vi "Accelerator_v2.002_small.vi"() -> ()   [LabVIEW 2013]
doc: "Acquire Accelerator Data"
uses:
  <instrlib>/niScope/Controls/niScope vertical coupling.ctl
  <instrlib>/niScope/Controls/niScope trigger slope.ctl
  <instrlib>/niScope/Controls/niScope trigger coupling.ctl
  <instrlib>/niScope/Controls/niScope trigger source.ctl
  Accelerator Measurement/Array_Defctl.ctl
  <vilib>/Utility/error.llb/DialogType.ctl
  <vilib>/Utility/miscctls.llb/LVPointTypeDef.ctl
  <vilib>/Utility/miscctls.llb/LVPositionTypeDef.ctl
  Public API/Dust_Event.ctl
  Public API/Signal.ctl
  Private/Role ID.ctl
  Private/Hardware ID.ctl
  Private/Estimate_source.ctl
  Functional Global Variables/Action Items.ctl
  <vilib>/Analysis/baseanly.llb/Mean (DBL).vi
  Private/PSU updated.vi
  <vilib>/addons/database/Connection.llb/Conn Execute.vi
  <vilib>/addons/database/Recordset.llb/Rec Fetch Recordset Data (R).vi
  <vilib>/addons/database/Recordset.llb/Rec Destroy - Connection.vi
  <instrlib>/niScope/Configure/Trigger/niScope Configure Trigger Edge.vi
  <instrlib>/niScope/Acquire/Fetch/niScope Multi Fetch Cluster.vi
  <vilib>/addons/database/_DB Variant To Data/Database Variant To Data.xnode
  <vilib>/Analysis/NI_AALBase.lvlib
  <vilib>/addons/database/NI_Database_API.lvlib
panel:
  in  "Trigger":enum32{"Edge"}(tab)
  in  "Trigger Source Edge 2":T1="2" caption="Source"
  in  "Trigger Source Edge":T1="0" caption="Source"
  in  "Coupling":T2=1 items=["AC"=0, "DC"=1, "HF Reject"=3, "LF Reject"=4, "AC Plus HF Reject"=1001]
  in  "Slope":T3 caption="Trigger Slope"
  in  "Level":dbl=1.0 caption="Trigger Level" step=0.001 format="%.3f"
  in  "Delay":dbl caption="Trigger Delay" format="%.4p"
  in  "Reference Position (%)":dbl=40.0 caption="Ref Position" format="%.1f"
  in  "Bandwidth":dbl=-1.0 format="%.2f"
  in  "Vertical Coupling":T4=1 items=["AC", "DC", "Ground"]
  in  "Probe Attenuation":dbl=1.0 format="%.1f"
  in  "Vertical Offset":dbl format="%.4f"
  in  "Vertical Range":dbl=5.0 caption="Vertical Range (V)" format="%.2f"
  out "Actual Sample Rate":dbl=10000000.0 format="%.0p"
  in  "Min Record Length":i32=100000 caption="Min. Record Length"
  in  "Min Sample Rate":dbl=80000000.0 caption="Min. Sample Rate" step=1000000.0 format="%.2p"
  out "Actual Record Length":i32=100000
  out "Mass":dbl format="%#_3g"
  in  "Write to Database?":bool=TRUE
  in  "Limit":dbl
  in  "Limit Triggers":bool
  out "Acquisition #":i32
  in  "WFM Tag":string="trace"
  in  "Location":string="G:\\default"
  in  "Write Raw File?":bool
  out "Saving Raw File...":path=path "G:/2012_06_13_verify_timestamp_labview/trace00000"
  out "?":cluster{dbl, dbl}(knob)={0.0549, 2.0} scale=10.0..0.01
  in  "Ideal Time (Cursor)":dbl=2.0 step=0.01 format="%_2f"
  out "Time Between Triggers":dbl
  out "Average Frequency":dbl format="%#_4g"
  out "output cluster":T5
  out "error out 4":errorcluster
  out "error out 3":errorcluster
  out "# elements in queue":i32
  out "Stop condition":bool=TRUE
  out "created path":path=path "G:/default"
  out "Numeric":i32=92364
  out "error out 2":errorcluster
  out "Calibration":dbl=24700000000000.0
  out "Array":T6=["Dev1", "Dev2"]
  out "Multi Plot 2":cluster{dbl[], dbl[]}(graph) caption="Multi Plot"
  in  "Acceleration Voltage (MV)":dbl=2.0 format="%_2g"
  out "Charge":dbl format="%#_3g"
  out "Velocity (Est.)":dbl format="%#_6f"
  out "Final Detector (CH3)":waveform(dbl)(graph)={"t0"=timestamp(0 s since 1904-01-01), "dt"=1e-07, "Y"=[]}
  out "Charge Detector/PSU gate (CH2)":waveform(dbl)(graph)={"t0"=timestamp(0 s since 1904-01-01), "dt"=1e-07, "Y"=[]}
  out "Velocity Detectors (CH0 & CH1)":waveform(dbl)[](graph)
  in  "stop":bool=TRUE
  out "error out":errorcluster={"status"=FALSE, "code"=0, "source"="No Error"} {"code" format="%.0x"}
  # "File Parameters"
  # "Error Handling"
  # "Trigger"
  # "Channel"
  # "Vertical"
  # "Horizontal"
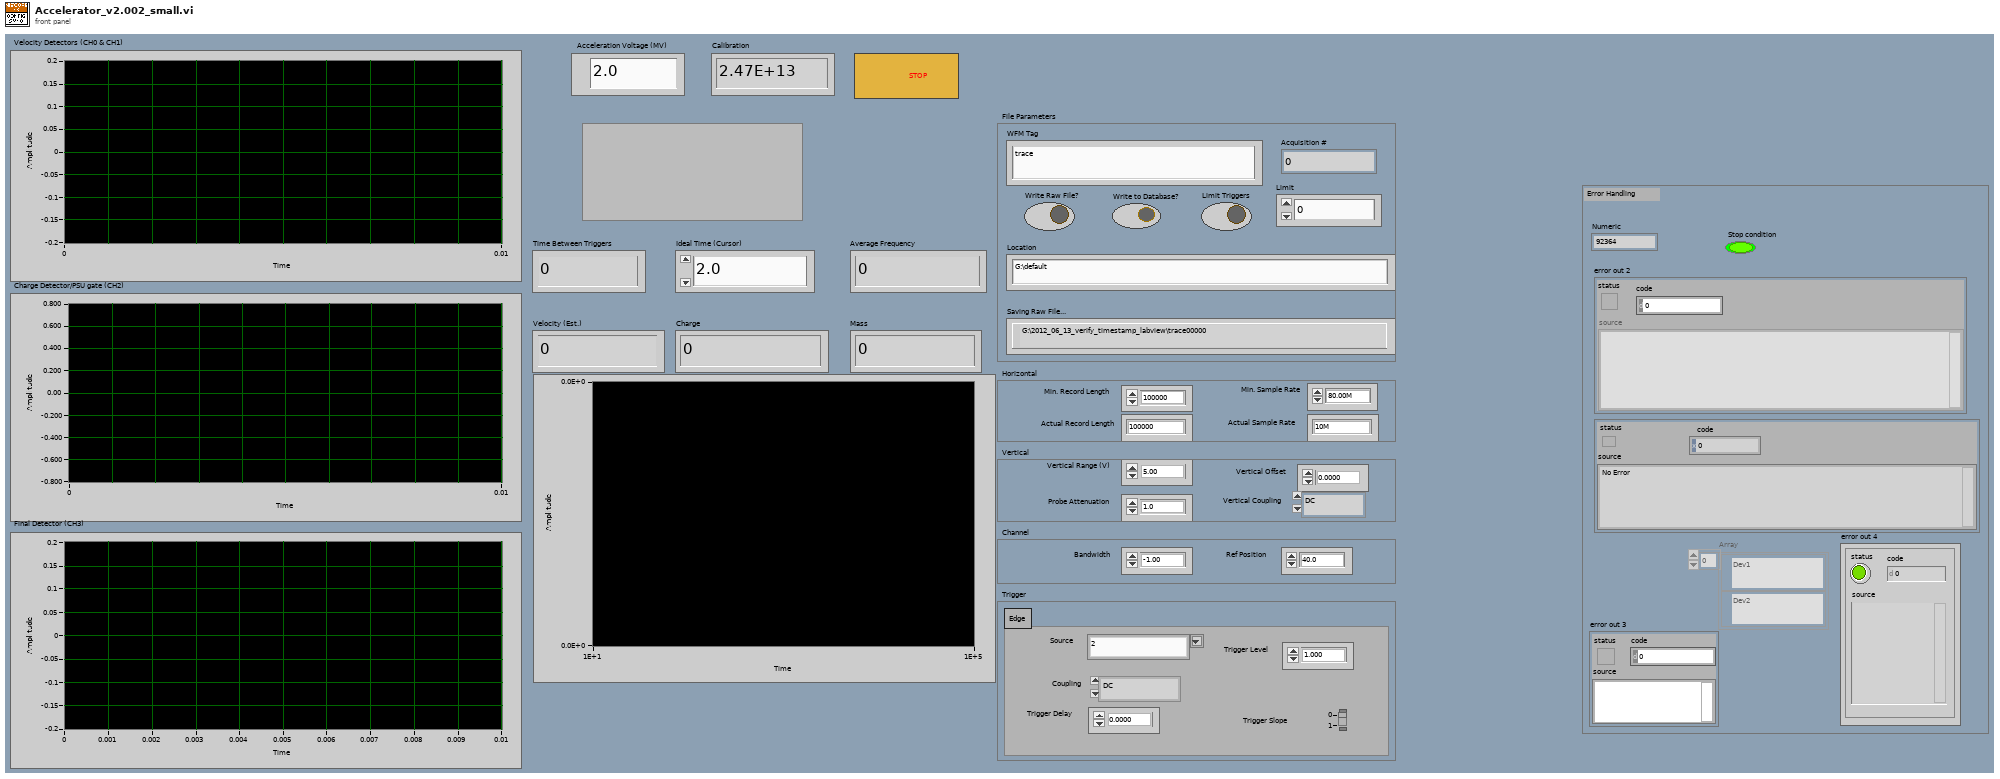
[diagram p1: front panel]
types:
  T1 = typedef "niScope trigger source.ctl" = string
  T2 = typedef "niScope trigger coupling.ctl" = u16
  T3 = typedef "niScope trigger slope.ctl" = i32
  T4 = typedef "niScope vertical coupling.ctl" = i32
  T5 = cluster{"File Path Control":path, "Array":waveform(dbl)[]}
  T6 = typedef "Array_Defctl.ctl" = refnum<k15>[]
  T7 = typedef "LVPointTypeDef.ctl" = cluster{"Horizontal":i16, "Vertical":i16}
  T8 = typedef "DialogType.ctl" = u16
  T9 = typedef "LVPositionTypeDef.ctl" = cluster{"Left":i32, "Top":i32}
  T10 = typedef "NI_Database_API.lvlib/Conn ObjectReference.ctl" = refnum<k1>
  T11 = typedef "NI_Database_API.lvlib/Rec ObjectReference.ctl" = refnum<k1>
  T12 = cluster{"Integer Timestamp":dbl, "Max Velocity":dbl, "Min Velocity":dbl}
  T13 = cluster{"first point time":dbl, "xIncrement":dbl, "Waveforms":dbl[]}[]
  T14 = typedef "Dust_Event.ctl" = cluster{"Time Stamp":timestamp, "Velocity":sgl, "Mass":sgl, "Charge":sgl, "Radius":sgl, "Array":T15[], "Dust Event ID":i64, "Passed_3rd_Detector":bool, "Estimate Source":T18, "Estimate Quality":sgl}
  T15 = typedef "Signal.ctl" = cluster{"Signal ID":i64, "Time Stamp":timestamp, "Dust Event ID":i64, "Role ID":T16, "Data":sgl[], "Signal Length":i32, "dt":sgl, "Offset":dbl, "Hardware ID":T17}
  T16 = typedef "Role ID.ctl" = enum16{"First_Detector", "Second_Detector", "Third_Detector", "LeCroy_CH1", "LeCroy_CH2", "LeCroy_CH3", "LeCroy_CH4", "PSU"}
  T17 = typedef "Hardware ID.ctl" = enum16{"Unknown", "CSA 1", "CSA 2", "CSA 3", "CSA 4", "CSA 5", "CSA 6"}
  T18 = typedef "Estimate_source.ctl" = i8
  T19 = typedef "Action Items.ctl" = enum16{"Initialize", "Get", "Set"}
  T20 = cluster{"relativeInitialX":dbl, "xIncrement":dbl, "wfm":dbl[]}[]
  T21 = cluster{"first point time":dbl, "xIncrement":dbl, "Waveforms":dbl[]}
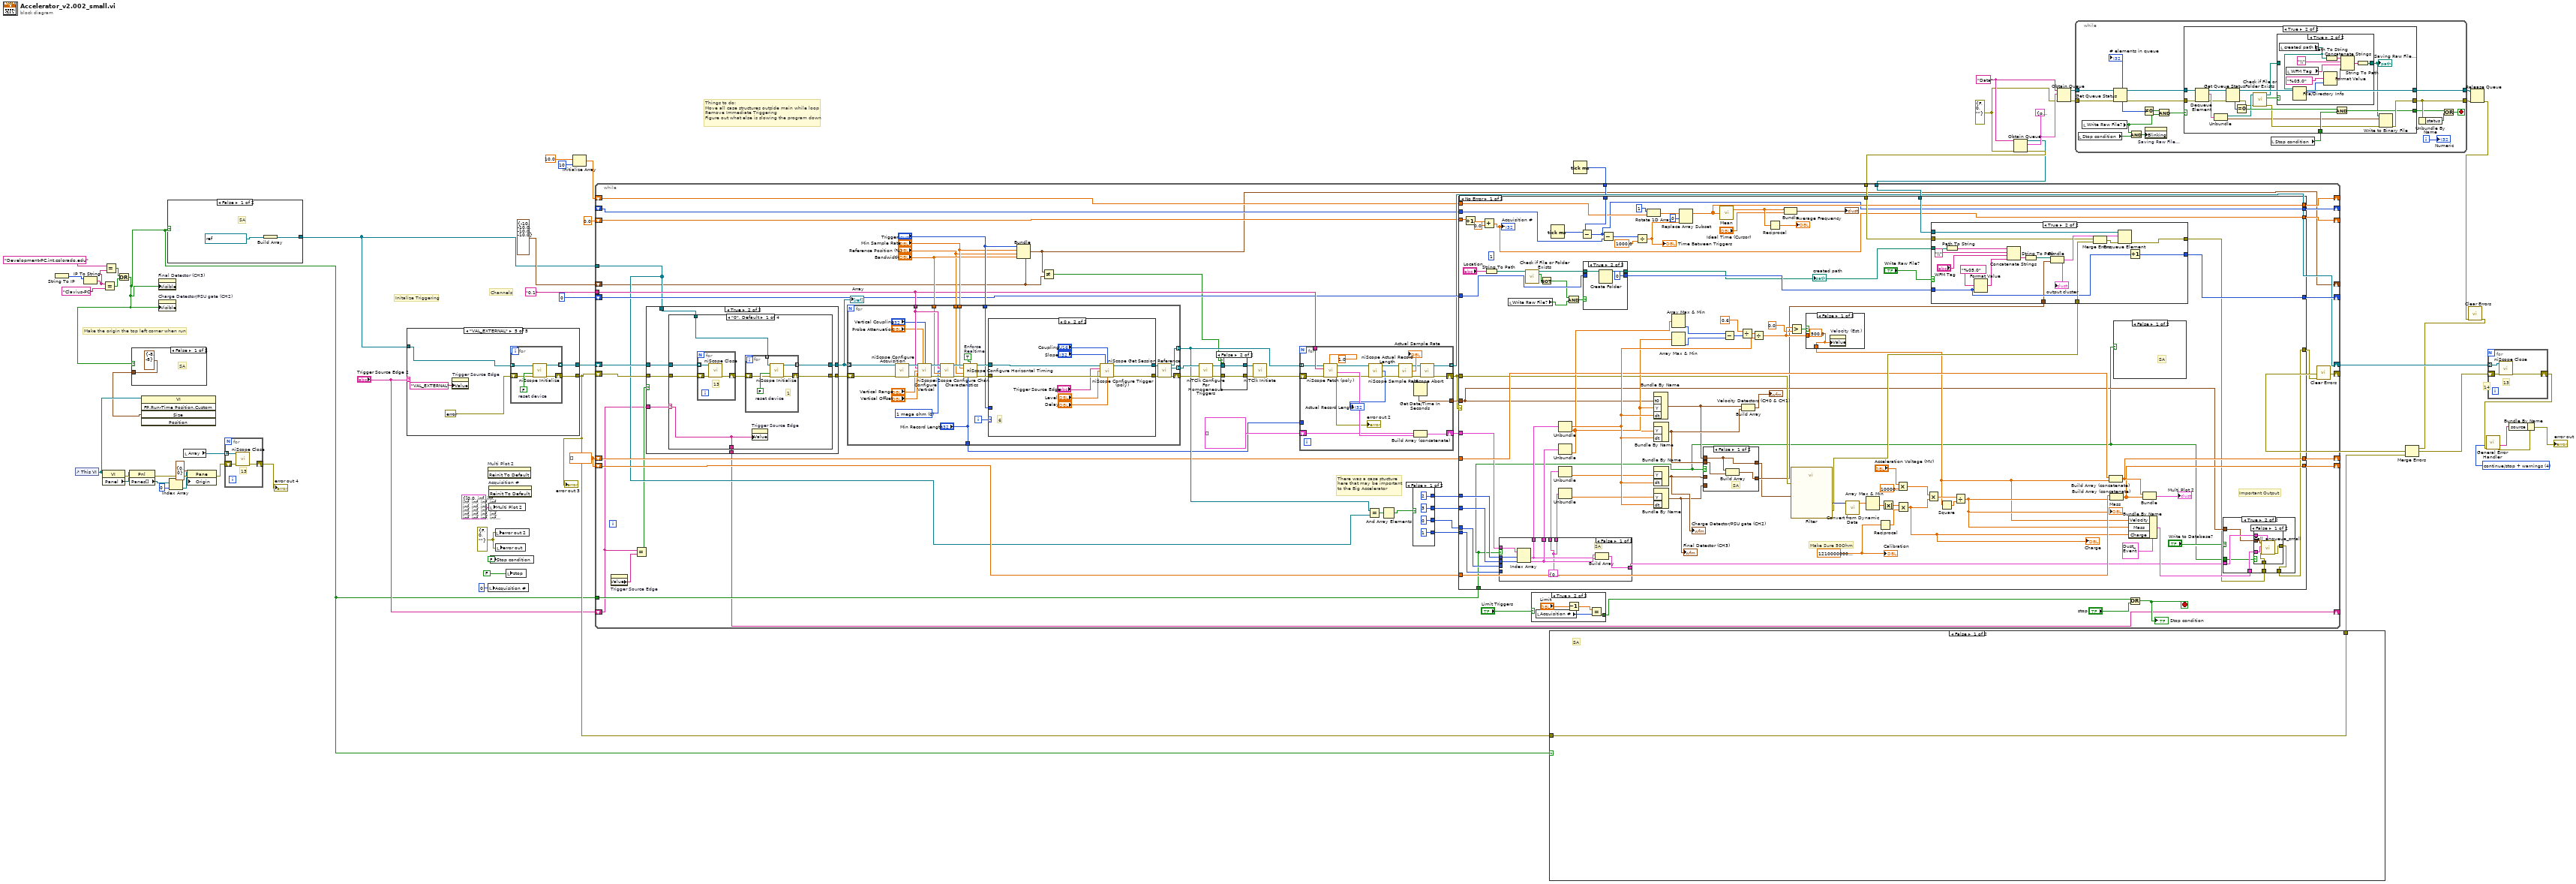
[diagram p0: block diagram]
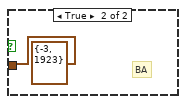
[diagram p2: hidden frame]
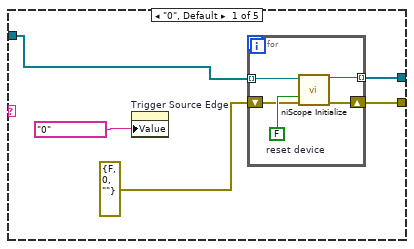
[diagram p3: hidden frame]
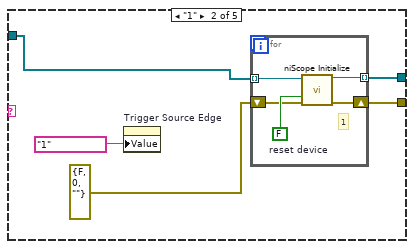
[diagram p4: hidden frame]
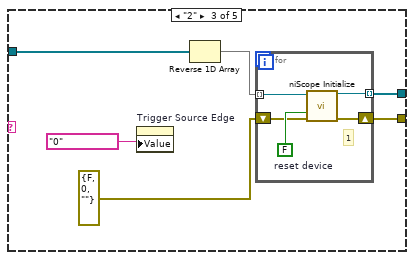
[diagram p5: hidden frame]
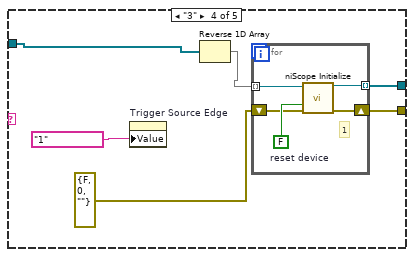
[diagram p6: hidden frame]
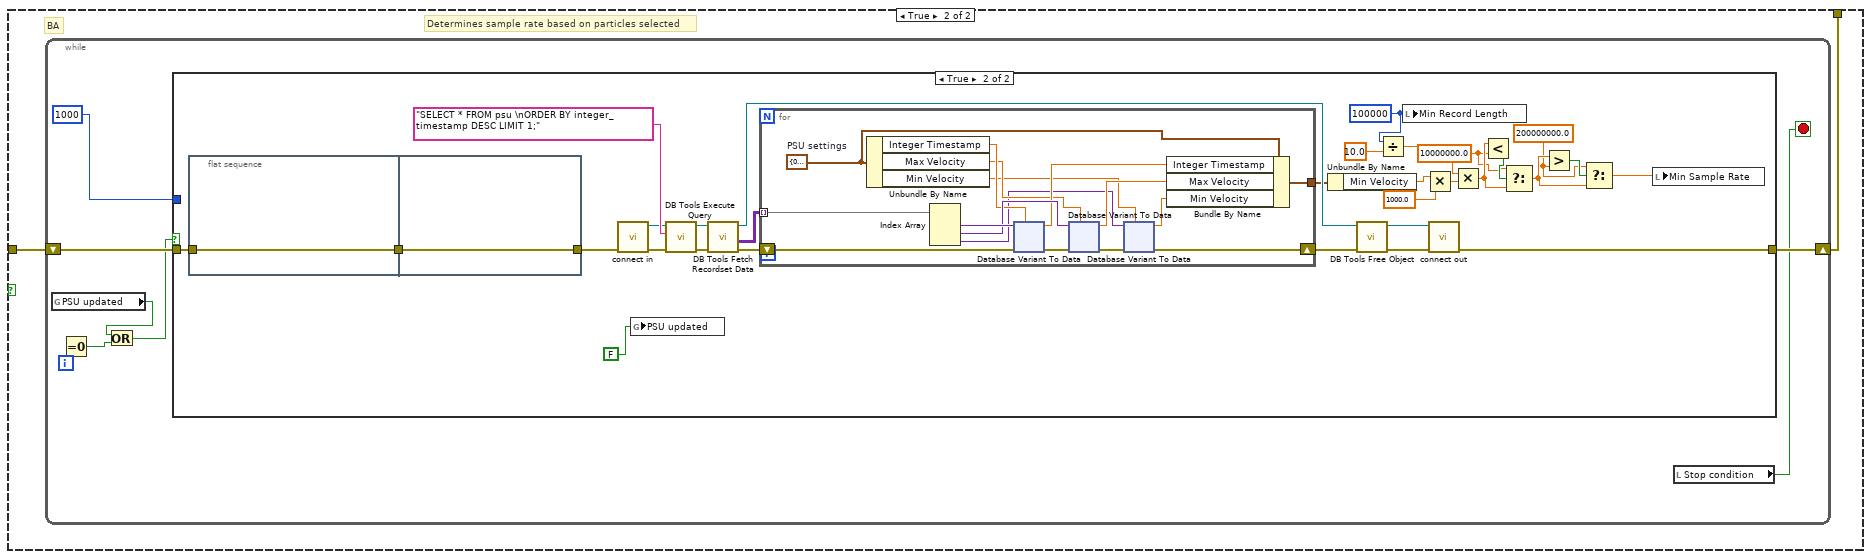
[diagram p7: hidden frame]
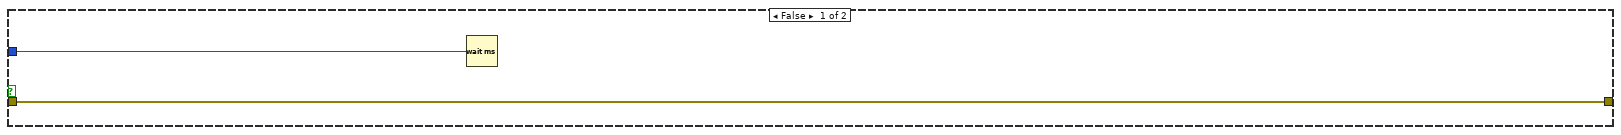
[diagram p8: hidden frame]
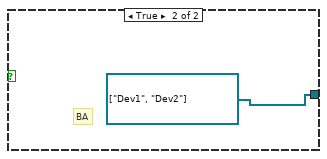
[diagram p9: hidden frame]
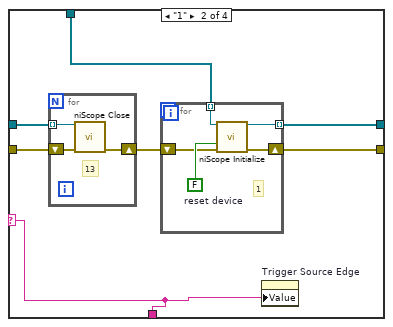
[diagram p11: hidden frame]
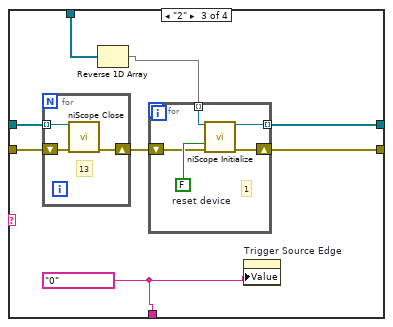
[diagram p12: hidden frame]
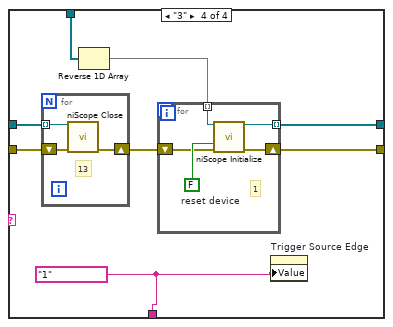
[diagram p13: hidden frame]
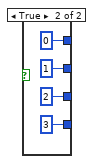
[diagram p14: hidden frame]
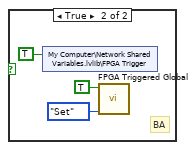
[diagram p16: hidden frame]
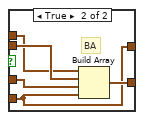
[diagram p17: hidden frame]
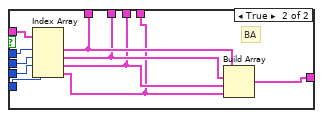
[diagram p18: hidden frame]
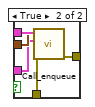
[diagram p20: hidden frame]
diagram:
  w23 = dbl[] []
  w30 = errorcluster {"status"=FALSE, "code"=0, "source"=""} ("error out")
  w35 = errorcluster {"status"=FALSE, "code"=0, "source"=""} ("error out")
  w36 = cluster{path, waveform(sgl)[]} {path "", []} ("output cluster")
  w37 = "Data" ("name (unnamed)")
  w28 = T8 4 items=["no dialog", "OK message", "continue or stop message", "OK message + warnings", "continue/stop + warnings"] ("type of dialog (OK msg:1)")
  # "Things to do:\nMove all case structures outside main while loop\nRemove Immediate Triggering\nFigure out what else is slowing the program down"
  # "Channels"
  # "Make the origin the top left corner when run"
  # "Initalize Triggering"
  # "14"
  n1 = String To IP() -> (0:w10:u32)  [unwired: 1 in]
  n2 = control-ref of="This VI"() -> (w3:refnum<vi>)
  n3 = IP To String(2:w10) -> (0:w5:string)  [unwired: 1 in]
  n4 = property class="VI"(reference=w3) -> (error out=w19:errorcluster, "Panel"=w18:refnum<vi>)  [unwired: 1 in, 1 out]
  n5 = Equal?(x=w5, y="Clavius-PC") -> (x = y?=w7:bool)
  n6 = Equal?(x="Development-PC.int.colorado.edu", y=w5) -> (x = y?=w6:bool)
  n7 = Or(x=w6, y=w7) -> (x .or. y?=w2:bool)
  n8 = property class="Pnl"(reference=w18, error in=w19) -> (error out=w17:errorcluster, "Panes[]"=w16:refnum<vi>[])  [unwired: 1 out]
  n9 = case shown="False" w2 {
    tunnel: [T9 {"Left"=-8, "Top"=-8} ("Position") T9 {"Left"=-3, "Top"=1923} ("Position")] -> w1
    frame False {
      # "SA"
    }
    frame True {
      # "BA"
    }
  }
  n10 = invoke class="VI" method="FP.Run-Time Position.Custom"(reference=w3, "Size"=w1) -> ()  [unwired: 3 in, 5 out]
  n11 = property on="Final Detector (CH3)" class="WFGraph (strict)"("Visible"=w2) -> ()  [unwired: 2 in, 2 out]
  n12 = property on="Charge Detector/PSU gate (CH2)" class="WFGraph (strict)"("Visible"=w2) -> ()  [unwired: 2 in, 2 out]
  n13 = case shown="False" w2 {
    tunnel: [w60 refnum<k15>[] ["Dev1", "Dev2"] ("Resources")] -> w11
    frame False {
      # "SA"
      n14 = Build Array(refnum<k15> "Dev5" ("resource name")) -> (w60:refnum<k15>[])
    }
    frame True {
      # "BA"
    }
  }
  n15 = Index Array(array=w16, index=0) -> (element=w14:refnum<vi>)
  n16 = local read "Array"() -> (w38:T6)
  n17 = property class="Pane"(reference=w14, error in=w17, "Origin"=T7 {"Horizontal"=0, "Vertical"=0}) -> (error out=w12:errorcluster)  [unwired: 1 out]
  n18 = for {
    tunnel: w38 -> [w63] mode=indexing
    shift-right: [w65] -> w33
    shift-left: w12 -> [w64]
    # "13"
    n19 = call <instrlib>:"niScope Close.vi"("instrument handle"=w63, "error in"=w64) -> ("error out"=w65:errorcluster)  [unwired: 13 in]
  }
  "error out 4" <- w33
  n20 = case shown="\"VAL_EXTERNAL\"" "Trigger Source Edge 2" {
    tunnel: [w70 w79 w90 w101 w112] -> w56
    tunnel: [w69 w78 w89 w100 w111] -> w21
    tunnel: w11 -> [w66 w76 w86 w97 w108]
    frame "0", Default {
      n21 = property on="Trigger Source Edge" class="CmbBox (strict)"("Value"=T1 "0" ("Trigger Source Edge")) -> ()  [unwired: 2 in, 2 out]
      n22 = for {
        tunnel: w66 -> [w74] mode=indexing
        tunnel: [w72] -> w70 mode=indexing
        shift-right: [w71] -> w69
        shift-left: errorcluster {"status"=FALSE, "code"=0, "source"=""} ("error out") -> [w73]
        w75 = FALSE  # reset device
        n23 = call <instrlib>:"niScope Initialize.vi"("resource name"=w74, "reset device"=w75, "error in"=w73) -> ("instrument handle"=w72:refnum<k15>, "error out"=w71:errorcluster)  [unwired: 11 in]
      }
    }
    frame "1" {
      n24 = property on="Trigger Source Edge" class="CmbBox (strict)"("Value"=T1 "1" ("Trigger Source Edge")) -> ()  [unwired: 2 in, 2 out]
      n25 = for {
        tunnel: w76 -> [w84] mode=indexing
        tunnel: [w82] -> w79 mode=indexing
        shift-right: [w81] -> w78
        shift-left: errorcluster {"status"=FALSE, "code"=0, "source"=""} ("error out") -> [w83]
        w85 = FALSE  # reset device
        # "1"
        n26 = call <instrlib>:"niScope Initialize.vi"("resource name"=w84, "reset device"=w85, "error in"=w83) -> ("instrument handle"=w82:refnum<k15>, "error out"=w81:errorcluster)  [unwired: 11 in]
      }
    }
    frame "2" {
      n27 = property on="Trigger Source Edge" class="CmbBox (strict)"("Value"=T1 "0" ("Trigger Source Edge")) -> ()  [unwired: 2 in, 2 out]
      n28 = Reverse 1D Array(array=w86) -> (reversed array=w87:refnum<k15>[])
      n29 = for {
        tunnel: w87 -> [w95] mode=indexing
        tunnel: [w93] -> w90 mode=indexing
        shift-right: [w92] -> w89
        shift-left: errorcluster {"status"=FALSE, "code"=0, "source"=""} ("error out") -> [w94]
        w96 = FALSE  # reset device
        # "1"
        n30 = call <instrlib>:"niScope Initialize.vi"("resource name"=w95, "reset device"=w96, "error in"=w94) -> ("instrument handle"=w93:refnum<k15>, "error out"=w92:errorcluster)  [unwired: 11 in]
      }
    }
    frame "3" {
      n31 = property on="Trigger Source Edge" class="CmbBox (strict)"("Value"=T1 "1" ("Trigger Source Edge")) -> ()  [unwired: 2 in, 2 out]
      n32 = Reverse 1D Array(array=w97) -> (reversed array=w98:refnum<k15>[])
      n33 = for {
        tunnel: w98 -> [w106] mode=indexing
        tunnel: [w104] -> w101 mode=indexing
        shift-right: [w103] -> w100
        shift-left: errorcluster {"status"=FALSE, "code"=0, "source"=""} ("error out") -> [w105]
        w107 = FALSE  # reset device
        # "1"
        n34 = call <instrlib>:"niScope Initialize.vi"("resource name"=w106, "reset device"=w107, "error in"=w105) -> ("instrument handle"=w104:refnum<k15>, "error out"=w103:errorcluster)  [unwired: 11 in]
      }
    }
    frame "VAL_EXTERNAL" {
      n35 = property on="Trigger Source Edge" class="CmbBox (strict)"("Value"=T1 "VAL_EXTERNAL" ("Trigger Source Edge")) -> ()  [unwired: 2 in, 2 out]
      n36 = for {
        tunnel: w108 -> [w116] mode=indexing
        tunnel: [w114] -> w112 mode=indexing
        shift-right: [w113] -> w111
        shift-left: errorcluster {"status"=FALSE, "code"=0, "source"=""} ("error out") -> [w115]
        w117 = FALSE  # reset device
        n37 = call <instrlib>:"niScope Initialize.vi"("resource name"=w116, "reset device"=w117, "error in"=w115) -> ("instrument handle"=w114:refnum<k15>, "error out"=w113:errorcluster)  [unwired: 11 in]
      }
    }
  }
  "error out 3" <- w21
  n38 = invoke on="Multi Plot 2" class="XYGraph (strict)" method="Reinit To Default"() -> ()  [unwired: 3 in, 3 out]
  n39 = local write "Acquisition #"(0 ("Acquisition #")) -> ()
  n40 = invoke on="Acquisition #" class="DigNum (strict)" method="Reinit To Default"() -> ()  [unwired: 3 in, 3 out]
  n41 = local write "Multi Plot 2"(cluster{dbl[], dbl[]} {[0.0, inf, inf, inf, inf, inf, inf, inf, inf, inf, inf, inf, inf, inf, inf, inf, inf, inf, inf, inf, inf, inf, inf, inf, inf, inf, inf, inf, inf, inf, inf, inf, inf, inf, inf, inf, inf, inf, inf, inf, inf], [0.0, 0.0, 0.0, 0.0, 0.0, 0.0, 0.0, 0.0, 0.0, 0.0, 0.0, 0.0, 0.0, 0.0, 0.0, 0.0, 0.0, 0.0, 0.0, 0.0, 0.0, 0.0, 0.0, 0.0, 0.0, 0.0, 0.0, 0.0, 0.0, 0.0, 0.0, 0.0, 0.0, 0.0, 0.0, 0.0, 0.0, 0.0, 0.0, 0.0, 0.0]} ("Multi Plot 2")) -> ()
  n42 = local write "Stop condition"(FALSE ("x .or. y?")) -> ()
  n43 = local write "error out 2"(w30) -> ()
  n44 = local write "error out"(w30) -> ()
  n45 = local write "stop"(FALSE ("stop")) -> ()
  n46 = Initialize Array(10.0 ("element"), 10 ("dimension size")) -> (w48:dbl[])
  n47 = case shown="False" w2 {
    tunnel: w21 -> [w118 w120]
    tunnel: [w118 w119] -> w20
    frame False {
      # "SA"
    }
    frame True {
      # "BA"
      # "Determines sample rate based on particles selected"
      n48 = while {
        shift-right: [w127] -> w119
        shift-left: w120 -> [w128]
        i -> [w126]
        stop <- w125 stop-if-true
        n49 = global read "PSU updated.vi" "PSU updated"() -> (w124:bool)
        n50 = Equal To 0?(x=w126) -> (x = 0?=w122:bool)
        n51 = Or(x=w124, y=w122) -> (x .or. y?=w123:bool)
        n52 = case shown="True" w123 {
          tunnel: w128 -> [w129 w159]
          tunnel: [w129 w158] -> w127
          tunnel: 1000 -> [w130 _]
          frame False {
            n53 = Wait (ms)(milliseconds to wait=w130) -> ()  [unwired: 1 out]
          }
          frame True {
            w132 = 200000000.0 ("y")
            w135 = 10000000.0 ("y")
            w142 = 100000 ("Min Record Length")
            n54 = flat-sequence {
              tunnel: [w161] -> w160
              tunnel: w159 -> [w161]
              tunnel: w160 -> [w162]
              tunnel: [w162] -> w145
              frame #0 {
              }
              frame #1 {
              }
            }
            n55 = call "connect in.vi"("error in (no error)"=w145) -> ("error out"=w149:errorcluster, "Database Connection"=w148:T10)  [unwired: 6 in, 1 out]
            n56 = global write "PSU updated.vi" "PSU updated"(FALSE ("PSU updated")) -> ()
            n57 = call-poly <vilib>:"DB Tools Execute Query.vi"("error in (no error)"=w149, "SQL query"="SELECT * FROM psu \nORDER BY integer_timestamp DESC LIMIT 1;", "connection reference"=w148) -> ("error out"=w151:errorcluster, "recordset reference"=w150:T11)  [unwired: 5 in]
            n58 = call-poly <vilib>:"DB Tools Fetch Recordset Data.vi"("error in (no error)"=w151, "recordset reference"=w150) -> ("error out"=w157:errorcluster, "recordset data"=w156:variant[][], "recordset reference out"=w152:T11)  [unwired: 3 in]
            n59 = for {
              tunnel: w156 -> [w178] mode=indexing
              shift-right: [w163] -> w146
              shift-left: w157 -> [w174]
              tunnel: [w173] -> w147
              w168 = T12 {"Integer Timestamp"=0.0, "Max Velocity"=0.0, "Min Velocity"=0.0}  # PSU settings
              n60 = Unbundle By Name(w168) -> ("Integer Timestamp"=w172:dbl, "Max Velocity"=w169:dbl, "Min Velocity"=w166:dbl)
              n61 = Index Array(array=w178) -> (element #1=w177:variant, element #2=w176:variant, element #3=w167:variant)  [unwired: 3 in]
              n62 = xnode "Database Variant To Data"("database variant"=w177, "error in"=w174, "type"=w172) -> ("data"=w171:dbl, "error out"=w175:errorcluster)
              n63 = xnode "Database Variant To Data"("database variant"=w176, "error in"=w175, "type"=w169) -> ("data"=w170:dbl, "error out"=w164:errorcluster)
              n64 = xnode "Database Variant To Data"("database variant"=w167, "error in"=w164, "type"=w166) -> ("data"=w165:dbl, "error out"=w163:errorcluster)
              n65 = Bundle By Name(cluster=w168, "Integer Timestamp"=w171, "Max Velocity"=w170, "Min Velocity"=w165) -> (w173:T12)
            }
            n66 = Unbundle By Name(w147) -> ("Min Velocity"=w141:dbl)
            n67 = call-poly <vilib>:"DB Tools Free Object.vi"("error in (no error)"=w146, "recordset reference"=w152) -> ("error out"=w153:errorcluster, "connection reference"=w154:T10)  [unwired: 8 in]
            n68 = Divide(x=w142, y=10.0) -> (x/y=w138:dbl)
            n69 = local write "Min Record Length"(w142) -> ()
            n70 = Multiply(x=w141, y=1000.0) -> (x*y=w139:dbl)
            n71 = call "connect out.vi"("error in (no error)"=w153, "connection reference"=w154) -> ("error out"=w158:errorcluster)  [unwired: 9 in]
            n72 = Multiply(x=w138, y=w139) -> (x*y=w136:dbl)
            n73 = Less?(x=w136, y=w135) -> (x < y?=w137:bool)
            n74 = Select(t=w135, s=w137, f=w136) -> (s? t:f=w134:dbl)
            n75 = Greater?(x=w134, y=w132) -> (0:w133:bool)
            n76 = Select(t=w132, s=w133, f=w134) -> (s? t:f=w131:dbl)
            n77 = local write "Min Sample Rate"(w131) -> ()
          }
        }
        n78 = local read "Stop condition"() -> (w125:bool)
      }
    }
  }
  n79 = Tick Count (ms)() -> (millisecond timer value=w51:u32)
  n80 = Obtain Queue(name (unnamed)=w37, element data type=w36, error in (no error)=w35) -> (queue out=w32:refnum<queue>, error out=w45:errorcluster)  [unwired: 2 in, 1 out]
  n81 = while {
    shift-right: [w293] -> w31
    shift-left: w21 -> [w298]
    shift-right: [w282] -> _
    shift-left: cluster{i32, dbl, dbl, dbl} {-10, -10.0, -10.0, -10.0} -> [w283]
    tunnel: w51 -> [w290]
    shift-right: [w288] -> _
    shift-left: w48 -> [w289]
    shift-right: [w287] -> _
    shift-left: _ -> [w291]
    shift-right: [w321] -> _
    shift-left: w23 -> [w302]
    shift-right: [w320] -> _
    shift-left: w23 -> [w319]
    tunnel: "0,1" ("Channel Name") -> [w318]
    shift-right: [w299] -> w46
    shift-left: w56 -> [w317]
    tunnel: w32 -> [w308]
    tunnel: w45 -> [w307]
    shift-right: [w306] -> _
    shift-left: 0 -> [w305]
    shift-right: [w285] -> _
    shift-left: 0.0 -> [w286]
    tunnel: w11 -> [w284]
    tunnel: w2 -> [w281]
    shift-right: [w276] -> _
    shift-left: "Trigger Source Edge 2" -> [w275]
    stop <- w297 stop-if-true
    # "There was a case stucture\nhere that may be important\nto the Big Accelerator"
    n82 = property on="Trigger Source Edge" class="CmbBox (strict)"() -> ("Value"=w277:T1)  [unwired: 2 in, 2 out]
    n83 = Equal?(x=w275, y=w277) -> (x = y?=w278:bool)
    n84 = case shown="True" w278 {
      tunnel: w317 -> [w336 w343]
      tunnel: [w335 w342] -> w316
      tunnel: [w336 w341] -> w315
      tunnel: w298 -> [w335 w340]
      tunnel: w284 -> [_ w339]
      tunnel: w275 -> [w334 w338]
      tunnel: [w334 w337] -> w276
      frame False {
      }
      frame True {
        n85 = case shown="\"0\", Default" w338 {
          selector: w338 -> [w344 w359 _ _]
          tunnel: w343 -> [w347 w362 w380 w394]
          tunnel: [w349 w364 w378 w395] -> w341
          tunnel: w340 -> [w346 w361 w379 w393]
          tunnel: [w348 w363 w377 w396] -> w342
          tunnel: w339 -> [w345 w360 w375 w392]
          tunnel: [w344 w359 w374 w390] -> w337
          frame "0", Default {
            n86 = for {
              tunnel: w347 -> [w351] mode=indexing
              shift-right: [w353] -> w350
              shift-left: w346 -> [w352]
              # "13"
              n87 = call <instrlib>:"niScope Close.vi"("instrument handle"=w351, "error in"=w352) -> ("error out"=w353:errorcluster)  [unwired: 13 in]
            }
            n88 = for {
              tunnel: [w357] -> w349 mode=indexing
              shift-right: [w356] -> w348
              shift-left: w350 -> [w354]
              tunnel: w345 -> [w355] mode=indexing
              w358 = FALSE  # reset device
              # "1"
              n89 = call <instrlib>:"niScope Initialize.vi"("resource name"=w355, "reset device"=w358, "error in"=w354) -> ("instrument handle"=w357:refnum<k15>, "error out"=w356:errorcluster)  [unwired: 11 in]
            }
            n90 = property on="Trigger Source Edge" class="CmbBox (strict)"("Value"=w344) -> ()  [unwired: 2 in, 2 out]
          }
          frame "1" {
            n91 = for {
              tunnel: w362 -> [w366] mode=indexing
              shift-right: [w368] -> w365
              shift-left: w361 -> [w367]
              # "13"
              n92 = call <instrlib>:"niScope Close.vi"("instrument handle"=w366, "error in"=w367) -> ("error out"=w368:errorcluster)  [unwired: 13 in]
            }
            n93 = for {
              tunnel: [w372] -> w364 mode=indexing
              shift-right: [w371] -> w363
              shift-left: w365 -> [w369]
              tunnel: w360 -> [w370] mode=indexing
              w373 = FALSE  # reset device
              # "1"
              n94 = call <instrlib>:"niScope Initialize.vi"("resource name"=w370, "reset device"=w373, "error in"=w369) -> ("instrument handle"=w372:refnum<k15>, "error out"=w371:errorcluster)  [unwired: 11 in]
            }
            n95 = property on="Trigger Source Edge" class="CmbBox (strict)"("Value"=w359) -> ()  [unwired: 2 in, 2 out]
          }
          frame "2" {
            w374 = T1 "0" ("Trigger Source Edge")
            n96 = for {
              tunnel: w380 -> [w382] mode=indexing
              shift-right: [w384] -> w381
              shift-left: w379 -> [w383]
              # "13"
              n97 = call <instrlib>:"niScope Close.vi"("instrument handle"=w382, "error in"=w383) -> ("error out"=w384:errorcluster)  [unwired: 13 in]
            }
            n98 = Reverse 1D Array(array=w375) -> (reversed array=w376:refnum<k15>[])
            n99 = for {
              tunnel: [w388] -> w378 mode=indexing
              shift-right: [w387] -> w377
              shift-left: w381 -> [w385]
              tunnel: w376 -> [w386] mode=indexing
              w389 = FALSE  # reset device
              # "1"
              n100 = call <instrlib>:"niScope Initialize.vi"("resource name"=w386, "reset device"=w389, "error in"=w385) -> ("instrument handle"=w388:refnum<k15>, "error out"=w387:errorcluster)  [unwired: 11 in]
            }
            n101 = property on="Trigger Source Edge" class="CmbBox (strict)"("Value"=w374) -> ()  [unwired: 2 in, 2 out]
          }
          frame "3" {
            w390 = T1 "1" ("Trigger Source Edge")
            n102 = for {
              tunnel: w394 -> [w398] mode=indexing
              shift-right: [w400] -> w397
              shift-left: w393 -> [w399]
              # "13"
              n103 = call <instrlib>:"niScope Close.vi"("instrument handle"=w398, "error in"=w399) -> ("error out"=w400:errorcluster)  [unwired: 13 in]
            }
            n104 = Reverse 1D Array(array=w392) -> (reversed array=w391:refnum<k15>[])
            n105 = for {
              tunnel: [w404] -> w395 mode=indexing
              shift-right: [w403] -> w396
              shift-left: w397 -> [w401]
              tunnel: w391 -> [w402] mode=indexing
              w405 = FALSE  # reset device
              # "1"
              n106 = call <instrlib>:"niScope Initialize.vi"("resource name"=w402, "reset device"=w405, "error in"=w401) -> ("instrument handle"=w404:refnum<k15>, "error out"=w403:errorcluster)  [unwired: 11 in]
            }
            n107 = property on="Trigger Source Edge" class="CmbBox (strict)"("Value"=w390) -> ()  [unwired: 2 in, 2 out]
          }
        }
      }
    }
    "Array" <- w315
    n108 = for {
      tunnel: w315 -> [w642] mode=indexing
      shift-right: [w620] -> w325
      shift-left: w316 -> [w641]
      tunnel: w318 -> [w633]
      tunnel: "Min Sample Rate" -> [w626]
      tunnel: "Trigger" -> [w625]
      tunnel: "Bandwidth" -> [w623]
      tunnel: "Reference Position (%)" -> [w622]
      tunnel: [w619] -> w310 mode=indexing
      tunnel: [w618] -> w322 mode=indexing
      tunnel: ["Min Record Length"] -> w309
      i -> [w627]
      w615 = u32 0 items=["1 mega ohm"] ("input impedance")
      w640 = TRUE  # Enforce Realtime
      n109 = call <instrlib>:"niScope Configure Acquisition.vi"("instrument handle"=w642, "error in"=w641) -> ("instrument handle out"=w638:refnum<k15>, "error out"=w639:errorcluster)  [unwired: 12 in]
      n110 = call <instrlib>:"niScope Configure Vertical.vi"("instrument handle"=w638, "probe attenuation"="Probe Attenuation", "vertical coupling"="Vertical Coupling", "channels"=w633, "vertical range"="Vertical Range", "vertical offset"="Vertical Offset", "error in"=w639) -> ("instrument handle out"=w637:refnum<k15>, "error out"=w636:errorcluster)  [unwired: 7 in]
      n111 = call <instrlib>:"niScope Configure Chan Characteristics.vi"("instrument handle"=w637, "channels"=w633, "input impedance"=w615, "maximum input frequency"=w623, "error in"=w636) -> ("instrument handle out"=w634:refnum<k15>, "error out"=w635:errorcluster)  [unwired: 9 in]
      n112 = call <instrlib>:"niScope Configure Horizontal Timing.vi"("instrument handle"=w634, "enforce realtime"=w640, "min sample rate"=w626, "reference position"=w622, "error in"=w635, "min record length"="Min Record Length") -> ("instrument handle out"=w629:refnum<k15>, "error out"=w630:errorcluster)  [unwired: 8 in]
      n113 = case shown="0" w627 {
        tunnel: w630 -> [w643 w653]
        tunnel: w629 -> [w644 w652]
        tunnel: [w644 w651] -> w617
        tunnel: [w643 w650] -> w621
        tunnel: w625 -> [_ _]
        frame 1, Default {
        }
        frame 0 {
          # "6"
          n114 = call-poly <instrlib>:"niScope Configure Trigger (poly).vi"("instrument handle"=w652, "trigger slope"="Slope", "trigger coupling"="Coupling", "trigger source"="Trigger Source Edge", "trigger level"="Level", "error in"=w653, "trigger delay"="Delay") -> ("instrument handle out"=w651:refnum<k15>, "error out"=w650:errorcluster)  [unwired: 7 in]
        }
      }
      n115 = call <instrlib>:"niScope Get Session Reference.vi"("instrument handle"=w617, "error in"=w621) -> ("instrument handle out"=w619:refnum<k15>, "session reference"=w618:refnum<k20>, "error out"=w620:errorcluster)  [unwired: 11 in]
    }
    n116 = Bundle(cluster=w283, "Trigger", "Min Sample Rate", "Reference Position (%)", "Bandwidth") -> (w282:cluster{i32, dbl, dbl, dbl})
    n117 = Not Equal?(x=w282, y=w283) -> (x != y?=w300:bool)
    n118 = call <instrlib>:"niTClk Configure For Homogeneous Triggers.vi"("error in (no error)"=w325, "sessions"=w322) -> ("error out"=w324:errorcluster, "sessions out"=w323:refnum<k20>[])  [unwired: 8 in]
    n119 = case shown="False" w300 {
      tunnel: [w612 w614] -> w332
      tunnel: [w611 w613] -> w331
      tunnel: w323 -> [w609 w614]
      tunnel: w324 -> [w610 w613]
      frame True {
        n120 = call <instrlib>:"niTClk Synchronize.vi"("error in (no error)"=w610, "sessions"=w609) -> ("error out"=w611:errorcluster, "sessions out"=w612:refnum<k20>[])  [unwired: 8 in]
      }
      frame False {
      }
    }
    n121 = call <instrlib>:"niTClk Initiate.vi"("error in (no error)"=w331, "sessions"=w332) -> ("error out"=w333:errorcluster)  [unwired: 8 in, 1 out]
    n122 = for {
      tunnel: w318 -> [w604]
      tunnel: w310 -> [w600] mode=indexing
      shift-right: [w608] -> w301
      shift-left: T13 [] ("Waveform Graph") -> [w602]
      shift-right: [w591] -> w294
      shift-left: w333 -> [w601]
      tunnel: w309 -> [_]
      tunnel: [w593] -> w299 mode=indexing
      tunnel: [w599] -> w303
      n123 = call-poly <instrlib>:"niScope Fetch (poly).vi"("timeout"=1.0 ("Timeout (s)"), "error in"=w601, "channels"=w604, "instrument handle"=w600) -> ("error out"=w595:errorcluster, "waveform"=w603:T20, "instrument handle out"=w596:refnum<k15>)  [unwired: 4 in, 1 out]
      "error out 2" <- w595
      n124 = call <instrlib>:"niScope Actual Record Length.vi"("instrument handle"=w596, "error in"=w595) -> ("instrument handle out"=w607:refnum<k15>, "actual record length"=→"Actual Record Length":i32, "error out"=w606:errorcluster)  [unwired: 11 in]
      n125 = call <instrlib>:"niScope Sample Rate.vi"("instrument handle"=w607, "error in"=w606) -> ("instrument handle out"=w594:refnum<k15>, "actual sample rate"=→"Actual Sample Rate":dbl, "error out"=w592:errorcluster)  [unwired: 11 in]
      n126 = Get Date/Time In Seconds() -> (seconds since 1Jan1904=w599:timestamp)
      n127 = Build Array (concatenate)(w602, w603) -> (w608:T20)
      n128 = call <instrlib>:"niScope Abort.vi"("instrument handle"=w594, "error in"=w592) -> ("instrument handle out"=w593:refnum<k15>, "error out"=w591:errorcluster)  [unwired: 12 in]
    }
    n129 = Equal?(x=w310, y=w284) -> (x = y?=w280:bool[])
    n130 = And Array Elements(Boolean array=w280) -> (logical AND=w279:bool)
    n131 = case shown="False" w279 {
      tunnel: [2 ("index") 0 ("index")] -> w314
      tunnel: [3 ("index") 1 ("index")] -> w313
      tunnel: [0 ("index") 2 ("index")] -> w312
      tunnel: [1 ("index") 3 ("index")] -> w311
      frame False {
      }
      frame True {
      }
    }
    n132 = case shown="No Error" w294 {
      tunnel: [w491 w583] -> w321
      tunnel: [w490 w584] -> w320
      tunnel: w319 -> [w489 w584]
      tunnel: w314 -> [w434 _]
      tunnel: w313 -> [w433 _]
      tunnel: w312 -> [w432 _]
      tunnel: w311 -> [w431 _]
      tunnel: w308 -> [w485 _]
      tunnel: w307 -> [w484 _]
      tunnel: [w480 w585] -> w306
      tunnel: w305 -> [w479 w585]
      tunnel: w303 -> [w440 _]
      tunnel: w302 -> [w470 w583]
      tunnel: w301 -> [w435 _]
      tunnel: w294 -> [w461 w582]
      tunnel: [w438 w582] -> w292
      tunnel: w291 -> [w445 w581]
      tunnel: w290 -> [w449 _]
      tunnel: w289 -> [w448 w580]
      tunnel: [w447 w580] -> w288
      tunnel: [w446 w581] -> w287
      tunnel: w286 -> [w442 w579]
      tunnel: [w441 w579] -> w285
      tunnel: w281 -> [w419 _]
      frame No Error {
        w487 = 12100000000000.0 ("x")
        (unwired) 1
        # "Important Output"
        # "Make Sure 50Ohm"
        n133 = Increment(x=w442) -> (x+1=w443:dbl)
        n134 = Add(x=w443, y=0.0) -> (x+y=w441:dbl)
        "Acquisition #" <- w441
        n135 = String To Path(string="Location") -> (path=w482:path)
        n136 = case shown="False" w419 {
          tunnel: w435 -> [w528 w538]
          tunnel: w434 -> [w527 w537]
          tunnel: w433 -> [w526 w536]
          tunnel: w432 -> [_ w535]
          tunnel: w431 -> [_ w534]
          tunnel: [w525 w533] -> w430
          tunnel: [w522 w529] -> w426
          tunnel: [w522 w530] -> w425
          tunnel: [w524 w531] -> w424
          tunnel: [w523 w532] -> w423
          frame False {
            w522 = T21 {"first point time"=0.0, "xIncrement"=0.0, "Waveforms"=[]} ("Waveforms")
            # "SA"
            n137 = Index Array(array=w528, index #1=w527, index #2=w526) -> (element #1=w523:T21, element #2=w524:T21)
            n138 = Build Array(w523, w524) -> (w525:T13)
          }
          frame True {
            # "BA"
            n139 = Index Array(array=w538, index #1=w537, index #2=w536, index #3=w535, index #4=w534) -> (element #1=w532:T21, element #2=w531:T21, element #3=w530:T21, element #4=w529:T21)
            n140 = Build Array(w532, w531, w530, w529) -> (w533:T13)
          }
        }
        n141 = local read "Write Raw File?"() -> (w414:bool)
        n142 = call <vilib>:"Check if File or Folder Exists.vi"("path"=w482) -> ("file or folder exists?"=w418:bool, "dup path"=w415:path)  [unwired: 8 in, 1 out]
        n143 = Not(x=w418) -> (.not. x?=w417:bool)
        n144 = Tick Count (ms)() -> (millisecond timer value=w454:u32)
        n145 = Unbundle(w423) -> ("xIncrement"=w475:dbl, "Waveforms"=w469:dbl[])  [unwired: 1 out]
        n146 = Unbundle(w424) -> ("Waveforms"=w468:dbl[])  [unwired: 2 out]
        n147 = Unbundle(w425) -> ("Waveforms"=w467:dbl[])  [unwired: 2 out]
        n148 = Unbundle(w426) -> ("Waveforms"=w466:dbl[])  [unwired: 2 out]
        n149 = And(x=w417, y=w414) -> (x .and. y?=w416:bool)
        n150 = Subtract(x=w454, y=w449) -> (x-y=w446:u32)
        n151 = case shown="True" w416 {
          tunnel: [w507 w510] -> w471
          tunnel: w415 -> [w507 w509]
          tunnel: w479 -> [w506 _]
          tunnel: [w506 0] -> w478
          frame False {
          }
          frame True {
            n152 = Create Folder(path (use dialog)=w509) -> (created path=w510:path)  [unwired: 2 in, 2 out]
          }
        }
        "created path" <- w471
        n153 = Subtract(x=w446, y=w445) -> (x-y=w455:u32)
        n154 = Divide(x=w455, y=1000.0) -> (x/y=w453:dbl)
        "Time Between Triggers" <- w453
        n155 = Rotate 1D Array(1:w448, 2:1 ("n")) -> (0:w458:dbl[])
        n156 = Bundle By Name("t0"=w440, "Y"=w469, "dt"=w475) -> (w420:waveform(dbl))  [unwired: 1 in]
        n157 = Bundle By Name("Y"=w468, "dt"=w475) -> (w428:waveform(dbl))  [unwired: 1 in]
        n158 = Bundle By Name("Y"=w467, "dt"=w475) -> (w429:waveform(dbl))  [unwired: 1 in]
        "Charge Detector/PSU gate (CH2)" <- w429
        n159 = Bundle By Name("Y"=w466, "dt"=w475) -> (w427:waveform(dbl))  [unwired: 1 in]
        "Final Detector (CH3)" <- w427
        n160 = Array Max & Min(array=w468) -> (min index (indices)=w477:i32)  [unwired: 3 out]
        n161 = Array Max & Min(array=w469) -> (min index (indices)=w476:i32)  [unwired: 3 out]
        n162 = Replace Array Subset(array=w458, new element=w453, index=0) -> (w447:dbl[])
        n163 = case shown="False" w419 {
          tunnel: w429 -> [_ w521]
          tunnel: w428 -> [w515 w520]
          tunnel: w420 -> [w514 w519]
          tunnel: w427 -> [_ w517]
          tunnel: [w516 w518] -> w422
          tunnel: [w514 w517] -> w421
          frame False {
            # "SA"
            n164 = Build Array(w514, w515) -> (w516:waveform(dbl)[])
          }
          frame True {
            # "BA"
            n165 = Build Array(w519, w520, w521, w517) -> (w518:waveform(dbl)[])
          }
        }
        n166 = call-poly <vilib>:"Mean.vi"("X"=w447) -> ("mean"=w452:dbl)  [unwired: 1 out]
        n167 = Subtract(x=w477, y=w476) -> (x-y=w504:i32)
        n168 = Divide(x=0.6, y=w504) -> (x/y=w502:dbl)
        n169 = Build Array(w420, w428) -> (→"Velocity Detectors (CH0 & CH1)":waveform(dbl)[])
        n170 = Divide(x=w502, y=w475) -> (x/y=w500:dbl)
        n171 = Reciprocal(x=w452) -> (1/x=→"Average Frequency":dbl)
        n172 = Bundle("mean"=w452, "Ideal Time (Cursor)"="Ideal Time (Cursor)") -> (→"?":cluster{"mean":dbl, "Ideal Time (Cursor)":dbl})  [unwired: 1 in]
        n173 = Greater?(x=w500, y=0.0 ("x")) -> (0:w501:bool)
        n174 = call "Filter"("error in (no error)"=w461, "Signal"=w421) -> ("error out"=w474:errorcluster, "Filtered Signal"=w488:dynamicdata)  [unwired: 8 in]
        n175 = case shown="False" w501 {
          tunnel: w500 -> [_ w578]
          tunnel: [w577 w578] -> w463
          frame False {
            w577 = 500.0 ("Velocity")
            n176 = property on="Velocity (Est.)" class="DigNum (strict)"("Value"=w577) -> ()  [unwired: 2 in, 2 out]
          }
          frame True {
            "Velocity (Est.)" <- w578
          }
        }
        n177 = call "Convert from Dynamic Data"("Dynamic Data Type"=w488) -> ("Array"=w498:dbl[])  [unwired: 3 in]
        n178 = Array Max & Min(array=w498) -> (min value=w497:dbl)  [unwired: 3 out]
        n179 = Reciprocal(x=w487) -> (1/x=w486:dbl)
        n180 = Absolute Value(x=w497) -> (abs(x)=w496:dbl)
        n181 = Multiply(x="Acceleration Voltage (MV)", y=1000000.0) -> (x*y=w472:dbl)
        n182 = Multiply(x=w496, y=w486) -> (x*y=w464:dbl)
        "Charge" <- w464
        n183 = Multiply(x=w472, y=w464) -> (x*y=w495:dbl)
        n184 = case shown="True" "Write Raw File?" {
          tunnel: w422 -> [_ w560]
          tunnel: [w557 w574] -> w437
          tunnel: w474 -> [w559 w572]
          tunnel: w485 -> [_ w561]
          tunnel: w484 -> [w558 w570]
          tunnel: w471 -> [_ w568]
          tunnel: [w556 w566] -> w480
          tunnel: w478 -> [w556 w565]
          frame False {
            n185 = Merge Errors(w558, w559) -> (w557:errorcluster)
          }
          frame True {
            n186 = Path To String(path=w568) -> (string=w563:string)
            n187 = Format Value(format string="%05.0", value (0)=w565) -> (output string=w567:string)  [unwired: 1 in]
            n188 = Concatenate Strings(w563, "\\" ("string"), "WFM Tag", w567) -> (w576:string)
            n189 = String To Path(string=w576) -> (path=w569:path)
            n190 = Bundle(w569, w560) -> (w571:cluster{path, waveform(dbl)[]})  [unwired: 1 in]
            "output cluster" <- w571
            n191 = Merge Errors(w570, w572) -> (w573:errorcluster)
            n192 = Enqueue Element(queue=w561, element=w571, error in (no error)=w573) -> (error out=w574:errorcluster)  [unwired: 1 in, 2 out]
            n193 = Increment(x=w565) -> (x+1=w566:i32)
          }
        }
        n194 = Square(x=w463) -> (x^2=w494:dbl)
        n195 = Divide(x=w495, y=w494) -> (x/y=w465:dbl)
        "Mass" <- w465
        n196 = Build Array (concatenate)(w470, w463) -> (w491:dbl[])
        n197 = Build Array (concatenate)(w489, w465) -> (w490:dbl[])
        n198 = case shown="False" w419 {
          frame False {
            # "SA"
          }
          frame True {
            # "BA"
            n199 = shared-variable "My Computer\\Network Shared Variables.lvlib\\FPGA Trigger"(TRUE ("FPGA Trigger")) -> ()  [unwired: 1 in, 1 out]
            n200 = call "FPGA Triggered Global.vi"("Action"=Action_Items."Set", "Input"=TRUE) -> ()  [unwired: 9 in, 1 out]
          }
        }
        n201 = Bundle By Name(cluster=T14 {"Time Stamp"=timestamp(0 s since 1904-01-01), "Velocity"=0.0, "Mass"=0.0, "Charge"=0.0, "Radius"=0.0, "Array"=[], "Dust Event ID"=0, "Passed_3rd_Detector"=FALSE, "Estimate Source"=0, "Estimate Quality"=0.0} ("Input Data"), "Velocity"=w463, "Mass"=w465, "Charge"=w464) -> (w439:T14)
        n202 = Bundle "Bundle"(w491, w490) -> (→"Multi Plot 2":cluster{dbl[], dbl[]})  [unwired: 1 in]
        n203 = case shown="True" "Write to Database?" {
          tunnel: w430 -> [_ w545]
          tunnel: w440 -> [_ w544]
          tunnel: w439 -> [_ w543]
          tunnel: [w539 w542] -> w438
          tunnel: w437 -> [w539 w541]
          tunnel: w419 -> [_ w540]
          frame False {
          }
          frame True {
            n204 = case shown="False" w540 {
              tunnel: w545 -> [w546 w555]
              tunnel: w544 -> [w547 w554]
              tunnel: w543 -> [w548 w553]
              tunnel: [w549 w552] -> w542
              tunnel: w541 -> [w550 w551]
              frame False {
                n205 = call "Call_enqueue_small.vi"("Waveform"=w546, "error in"=w550, "Input Data"=w548, "seconds since 1Jan1904"=w547) -> ("error IO"=w549:errorcluster)  [unwired: 7 in]
              }
              frame True {
                n206 = call "Call_enqueue.vi"("Waveform"=w555, "error in"=w551, "Input Data"=w553, "seconds since 1Jan1904"=w554) -> ("error IO"=w552:errorcluster)  [unwired: 7 in]
              }
            }
          }
        }
        "Calibration" <- w487
      }
      frame Error {
      }
    }
    n207 = case shown="True" "Limit Triggers" {
      tunnel: [FALSE w589] -> w296
      frame False {
      }
      frame True {
        n208 = local read "Acquisition #"() -> (w588:i32)
        n209 = Decrement(x="Limit") -> (x-1=w587:dbl)
        n210 = Equal?(x=w587, y=w588) -> (x = y?=w589:bool)
      }
    }
    n211 = Or(x=w296, y="stop") -> (x .or. y?=w297:bool)
    "Stop condition" <- w297
    n212 = call <vilib>:"Clear Errors.vi"("error in (no error)"=w292) -> ("error out"=w293:errorcluster)  [unwired: 6 in]
  }
  n213 = Obtain Queue(name (unnamed)=w37, element data type=w36, error in (no error)=w35) -> (queue out=w43:refnum<queue>, error out=w42:errorcluster)  [unwired: 2 in, 1 out]
  n214 = while {
    tunnel: w43 -> [w661]
    tunnel: w42 -> [w654]
    tunnel: [w670] -> w41
    tunnel: [w668] -> w40
    i -> [w664]
    stop <- w667 stop-if-true
    n215 = local read "Stop condition"() -> (w656:bool)
    n216 = local read "Write Raw File?"() -> (w658:bool)
    n217 = Get Queue Status(queue=w661, error in (no error)=w654) -> (queue out=w655:refnum<queue>, error out=w662:errorcluster, # elements in queue=w660:i32)  [unwired: 1 in, 5 out]
    "# elements in queue" <- w660
    n218 = And(x=w658, y=w656) -> (x .and. y?=w669:bool)
    n219 = Not Equal To 0?(x=w660) -> (x != 0?=w659:bool)
    n220 = property on="Saving Raw File..." class="Path"("Blinking"=w669) -> ()  [unwired: 2 in, 2 out]
    n221 = And(x=w659, y=w658) -> (x .and. y?=w663:bool)
    n222 = local read "Stop condition"() -> (w657:bool)
    n223 = case shown="True" w663 {
      tunnel: w655 -> [w674 w693]
      tunnel: [w672 w691] -> w668
      tunnel: [w673 w689] -> w670
      tunnel: w657 -> [w675 w688]
      tunnel: [w675 w685] -> w665
      tunnel: w662 -> [w671 w681]
      frame False {
        n224 = Flush Queue(queue=w674, error in (no error)=w671) -> (queue out=w673:refnum<queue>, error out=w672:errorcluster)  [unwired: 1 out]
      }
      frame True {
        n225 = Dequeue Element(queue=w693, error in (no error)=w681) -> (queue out=w690:refnum<queue>, element=w692:cluster{path, waveform(sgl)[]}, error out=w679:errorcluster)  [unwired: 1 in, 1 out]
        n226 = Unbundle(w692) -> (w680:path, w676:waveform(sgl)[])
        n227 = Get Queue Status(queue=w690, error in (no error)=w679) -> (queue out=w689:refnum<queue>, error out=w678:errorcluster, # elements in queue=w687:i32)  [unwired: 1 in, 5 out]
        n228 = Equal To 0?(x=w687) -> (x = 0?=w686:bool)
        n229 = call <vilib>:"Check if File or Folder Exists.vi"("error in (no error)"=w678, "path"=w680) -> ("error out"=w677:errorcluster, "file or folder exists?"=w684:bool, "dup path"=w683:path)  [unwired: 7 in]
        n230 = case shown="True" w684 {
          tunnel: w683 -> [w694 _]
          tunnel: [w694 w700] -> w682
          frame False {
          }
          frame True {
            n231 = local read "created path"() -> (w697:path)
            n232 = local read "WFM Tag"() -> (w702:string)
            n233 = File/Directory Info(path=w697) -> (size=w698:i64)  [unwired: 1 in, 6 out]
            n234 = Format Value(format string="%05.0", value (0)=w698) -> (output string=w701:string)  [unwired: 1 in]
            n235 = Path To String(path=w697) -> (string=w695:string)
            n236 = Concatenate Strings(w695, "\\" ("string"), w702, w701) -> (w699:string)
            n237 = String To Path(string=w699) -> (path=w700:path)
          }
        }
        "Saving Raw File..." <- w682
        n238 = And(x=w686, y=w688) -> (x .and. y?=w685:bool)
        n239 = Write to Binary File(file (use dialog)=w682, data=w676, error in=w677) -> (error out=w691:errorcluster)  [unwired: 3 in, 2 out]
      }
    }
    n240 = Unbundle By Name(w668) -> ("status"=w666:bool)
    n241 = Or(x=w665, y=w666) -> (x .or. y?=w667:bool)
    "Numeric" <- w664
  }
  n242 = Release Queue(queue=w41, error in (no error)=w40) -> (error out=w26:errorcluster)  [unwired: 1 in, 2 out]
  n243 = call <vilib>:"Clear Errors.vi"("error in (no error)"=w26) -> ("error out"=w25:errorcluster)  [unwired: 6 in]
  n244 = Merge Errors(w25, w31, w20) -> (w27:errorcluster)
  n245 = for {
    tunnel: w46 -> [w704] mode=indexing
    shift-right: [w706] -> w57
    shift-left: w27 -> [w705]
    # "13"
    n246 = call <instrlib>:"niScope Close.vi"("instrument handle"=w704, "error in"=w705) -> ("error out"=w706:errorcluster)  [unwired: 13 in]
  }
  n247 = call <vilib>:"General Error Handler.vi"("type of dialog (OK msg:1)"=w28, "error in (no error)"=w57) -> ("message"=w53:string, "error out"=w55:errorcluster)  [unwired: 9 in, 3 out]
  n248 = Bundle By Name(cluster=w55, "source"=w53) -> (→"error out":errorcluster)
